vi "Configure Chan Output.vi"(4 "Adjustable (5 Volts)":dbl=5.0 format="%.3p", 6 "Level (TTL)":T1(ring), 7 "Channel (1:Chan A)":i32(ring)=1 items=["Channel A"=1, "Channel B"=2, "Channel C"=3, "Channel D"=4, "Channel E"=5, "Channel F"=6, "Channel G"=7, "Channel H"=8], 8 "error in (no error)":errorcluster, 9 "MUX Value (-1)":i32=-1, 10 "Polarity (F:Normal)":bool, 11 "VISA resource name":refnum<visa-resource-name>) -> (0 "error out":errorcluster, 3 "VISA resource name out":refnum<visa-resource-name>)   [LabVIEW 2013, in "Berkeley Nucleonics 500 Series.lvlib"]
doc: "This VI is used to configure the output polarity and level of a channel.\n\nThe \"Adjustable\" parameter is only updated when operating in the \"Adjustable\" mode."
uses:
  Berkeley Nucleonics 500 Series.lvlib
panel:
  # "Note:\nThe \"Adjustable\" parameter is only updated when operating in the \"Adjustable\" level."
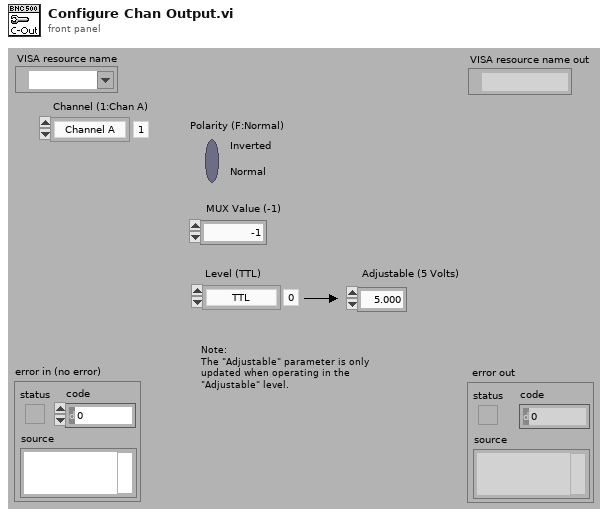
[diagram p1: front panel]
types:
  T1 = enum16{"TTL", "Adjustable", "35 Volt", "Optical"}
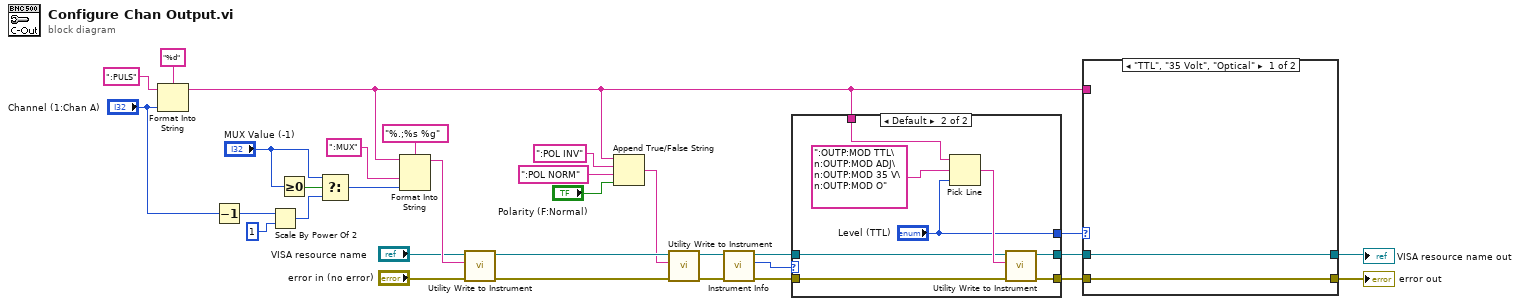
[diagram p0: block diagram]
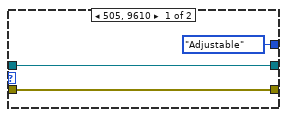
[diagram p2: hidden frame]
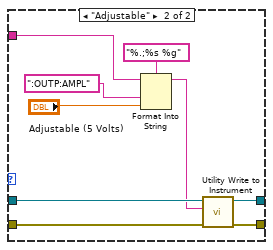
[diagram p3: hidden frame]
diagram:
  n1 = Format Into String(format string="%d", initial string=":PULS", "Channel (1:Chan A)") -> (resulting string=w8:string)  [unwired: 1 in, 1 out]
  n2 = Decrement(x="Channel (1:Chan A)") -> (x-1=w26:i32)
  n3 = Scale By Power Of 2(n=w26, x=1) -> (x*2^n=w24:i32)
  n4 = Greater Or Equal To 0?(x="MUX Value (-1)") -> (x >= 0?=w7:bool)
  n5 = Select(t="MUX Value (-1)", s=w7, f=w24) -> (s? t:f=w21:i32)
  n6 = Format Into String(format string="%.;%s %g", initial string=w8, ":MUX", w21) -> (resulting string=w20:string)  [unwired: 1 in, 1 out]
  n7 = call "Utility Write to Instrument.vi"("error in (no error)"="error in (no error)", "Write Buffer"=w20, "VISA resource name"="VISA resource name") -> ("error out"=w17:errorcluster, "VISA resource name out"=w16:refnum<visa-resource-name>)  [unwired: 6 in, 1 out]
  n8 = Append True/False String(1:"Polarity (F:Normal)", 2:":POL NORM", 3:":POL INV", 4:w8) -> (0:w13:string)
  n9 = call "Utility Write to Instrument.vi"("error in (no error)"=w17, "Write Buffer"=w13, "VISA resource name"=w16) -> ("error out"=w3:errorcluster, "VISA resource name out"=w4:refnum<visa-resource-name>)  [unwired: 6 in, 1 out]
  n10 = call "Instrument Info.vi"("error in (no error)"=w3, "VISA resource name"=w4) -> ("error out"=w2:errorcluster, "Instr Model"=w1:u32, "VISA resource name out"=w5:refnum<visa-resource-name>)  [unwired: 6 in, 1 out]
  n11 = case shown="Default" w1 {
    tunnel: [enum16{"TTL", "Adjustable", "35 Volt"}."Adjustable" ("Level (TTL)") "Level (TTL)"] -> w30
    tunnel: w5 -> [w34 w40]
    tunnel: w2 -> [w33 w39]
    tunnel: [w34 w38] -> w29
    tunnel: [w33 w37] -> w28
    tunnel: w8 -> [_ w36]
    frame 505, 9610 {
    }
    frame Default {
      n12 = Pick Line(string ("")=w36, multi-line string=":OUTP:MOD TTL\n:OUTP:MOD ADJ\n:OUTP:MOD 35 V\n:OUTP:MOD O", line index="Level (TTL)") -> (output string=w41:string)
      n13 = call "Utility Write to Instrument.vi"("error in (no error)"=w39, "Write Buffer"=w41, "VISA resource name"=w40) -> ("error out"=w37:errorcluster, "VISA resource name out"=w38:refnum<visa-resource-name>)  [unwired: 6 in, 1 out]
    }
  }
  n14 = case shown="\"TTL\", \"35 Volt\", \"Optical\"" w30 {
    tunnel: w8 -> [_ w52]
    tunnel: [w44 w47] -> w14
    tunnel: w29 -> [w44 w50]
    tunnel: [w43 w46] -> w15
    tunnel: w28 -> [w43 w51]
    frame "TTL", "35 Volt", "Optical" {
    }
    frame "Adjustable" {
      n15 = Format Into String(format string="%.;%s %g", initial string=w52, ":OUTP:AMPL", "Adjustable (5 Volts)") -> (resulting string=w49:string)  [unwired: 1 in, 1 out]
      n16 = call "Utility Write to Instrument.vi"("error in (no error)"=w51, "Write Buffer"=w49, "VISA resource name"=w50) -> ("error out"=w46:errorcluster, "VISA resource name out"=w47:refnum<visa-resource-name>)  [unwired: 6 in, 1 out]
    }
  }
  "error out" <- w15
  "VISA resource name out" <- w14
